vi "Scale_ADC Data.vi"(8 "error in (no error)":errorcluster, 11 "DAQ_Device in":refnum<class "RS232_Device.lvclass">) -> (0 "error out":errorcluster, 3 "DAQ_Device out":refnum<class "RS232_Device.lvclass">)   [LabVIEW 2023, in "RS232_Device.lvclass"]
uses:
  RS232_Device.lvclass
  DAQ Device_ChannelConfiguration.ctl
panel:
  in  "ADC/Register Value":u32
  in  "input cluster":T1={"Name"="", "InputType"=enum."Voltage (+/- 10V)", "UL"=0.0, "LL"=0.0, "GAIN"=0.0, "OFFSET"=0.0, "FACTOR"=0.0}
  out "output variable":dbl
  out "InRange?":bool
  out "Value":dbl
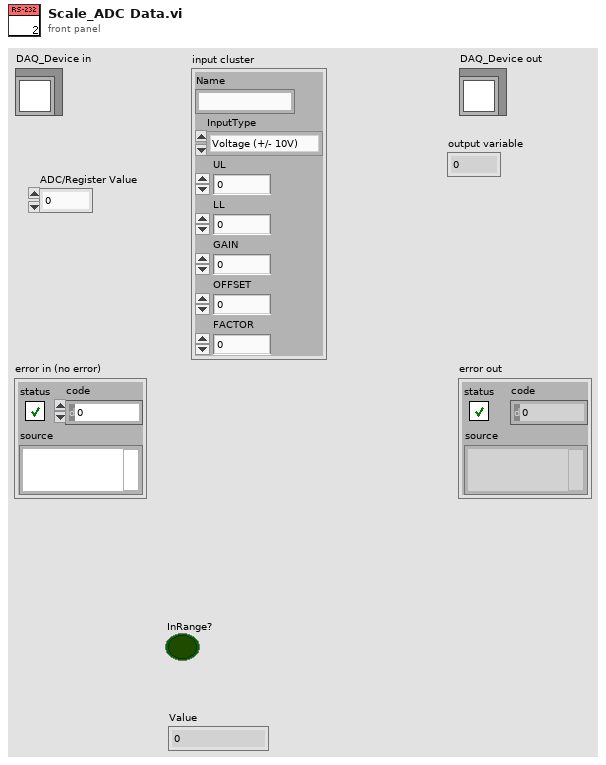
[diagram p1: front panel]
types:
  T1 = typedef "DAQ Device_ChannelConfiguration.ctl" = cluster{"Name":string, "InputType":enum16{"MB Register", "Current (4-20 mA)", "Current (0-20 mA)", "Voltage (+/- 10V)"}, "UL":dbl, "LL":dbl, "GAIN":dbl, "OFFSET":dbl, "FACTOR":dbl}
  T2 = enum16{"MB Register", "Current (4-20 mA)", "Current (0-20 mA)", "Voltage (+/- 10V)"}
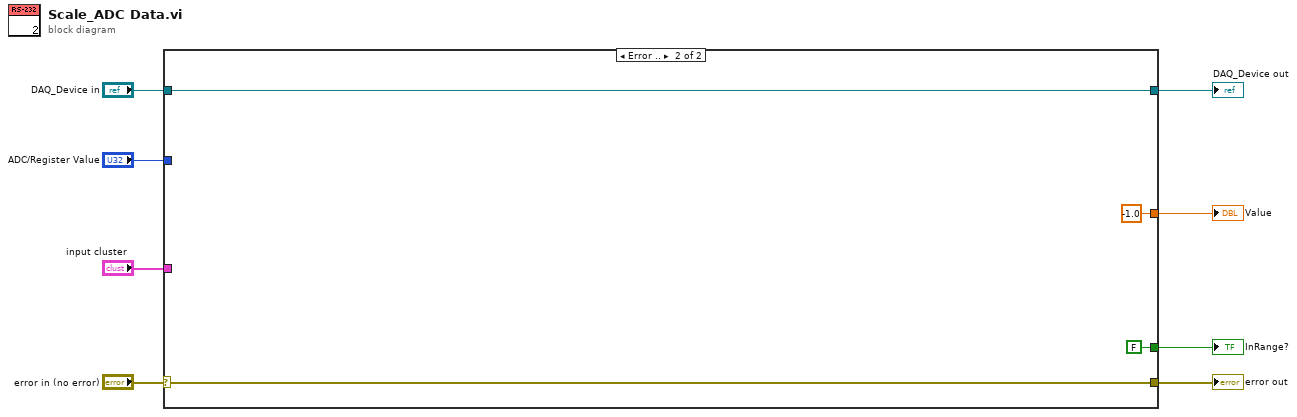
[diagram p0: block diagram]
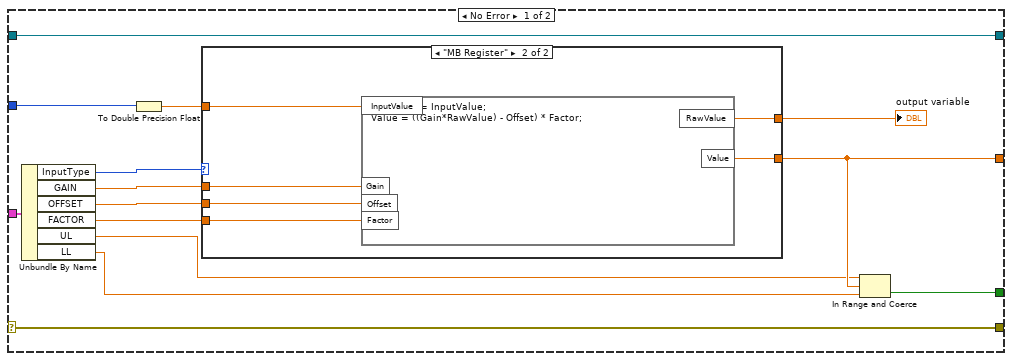
[diagram p2: hidden frame]
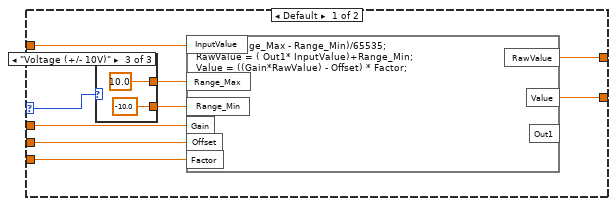
[diagram p3: hidden frame]
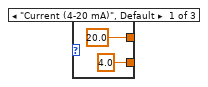
[diagram p4: hidden frame]
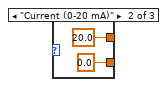
[diagram p5: hidden frame]
diagram:
  n1 = case shown="Error .." "error in (no error)" {
    selector: "error in (no error)" -> [w9 w45]
    tunnel: [w18 -1.0 ("Value")] -> w8
    tunnel: [w15 FALSE] -> w7
    tunnel: "input cluster" -> [w13 _]
    tunnel: "ADC/Register Value" -> [w12 _]
    tunnel: [w10 w46] -> w2
    tunnel: "DAQ_Device in" -> [w10 w46]
    tunnel: [w9 w45] -> w1
    frame No Error {
      n2 = Unbundle By Name(w13) -> ("InputType"=w14:T2, "GAIN"=w22:dbl, "OFFSET"=w21:dbl, "FACTOR"=w20:dbl, "UL"=w16:dbl, "LL"=w17:dbl)
      n3 = To Double Precision Float(number=w12) -> (double precision float=w11:dbl)
      n4 = case shown="\"MB Register\"" w14 {
        selector: w14 -> [w24 _]
        tunnel: w22 -> [w31 w43]
        tunnel: w21 -> [w30 w42]
        tunnel: w20 -> [w29 w41]
        tunnel: [w26 w40] -> w19
        tunnel: [w25 w39] -> w18
        tunnel: w11 -> [w23 w38]
        frame Default {
          n5 = case shown="\"Voltage (+/- 10V)\"" w24 {
            tunnel: [4.0 ("y") 0.0 ("y") -10.0 ("y")] -> w27
            tunnel: [20.0 ("y") 20.0 ("y") 10.0 ("y")] -> w28
            frame "Current (4-20 mA)", Default {
            }
            frame "Current (0-20 mA)" {
            }
            frame "Voltage (+/- 10V)" {
            }
          }
          n6 = formula code="Out1=(Range_Max - Range_Min)/65535;\nRawValue = ( Out1* InputValue)+Range_Min;\nValue = ((Gain*RawValue) - Offset) * Factor;"("Gain"=w31, "Offset"=w30, "Factor"=w29, "Range_Min"=w27, "Range_Max"=w28, "InputValue"=w23) -> ("Value"=w25:dbl, "RawValue"=w26:dbl)  [unwired: 1 out]
        }
        frame "MB Register" {
          n7 = formula code="RawValue = InputValue;\nValue = ((Gain*RawValue) - Offset) * Factor;"("Gain"=w43, "Offset"=w42, "Factor"=w41, "InputValue"=w38) -> ("Value"=w39:dbl, "RawValue"=w40:dbl)
        }
      }
      "output variable" <- w19
      n8 = In Range and Coerce(upper limit=w16, x=w18, lower limit=w17) -> (In Range?=w15:bool)  [unwired: 1 out]
    }
    frame Error {
    }
  }
  "error out" <- w1
  "DAQ_Device out" <- w2
  "Value" <- w8
  "InRange?" <- w7
